vi "check_run_settings_dialog.vi"(0 "Enable":bool=TRUE, 2 "Current Run Settings":T1={"Operator"="", "Sample (or CRM) ID"="", "Sample Temp"=0.0, "Salinity"=0.0, "Sample Units"=FALSE, "Sample Size"=0.0, "Operation Mode"=TRUE}, 5 "error in (no error)":errorcluster) -> (15 "New Run Settings":T1={"Operator"="", "Sample (or CRM) ID"="", "Sample Temp"=0.0, "Salinity"=0.0, "Sample Units"=FALSE, "Sample Size"=0.0, "Operation Mode"=TRUE}, 18 "OK":bool, 19 "error out":errorcluster)   [LabVIEW 2010]
doc: "Displays a standard dialog box that prompts users to enter information, such as a user name and password.\n--------------------\n\nThis Express VI is configured as follows:\n\nMessage to Display to the User:\nThe inputs are:"
panel:
  out "String":string
  in  "Cancel":bool
  in  "OK2":bool
  in  "OK1":bool
  # "Please verify that the following settings are correct and update them if need be (especially Operation Mode and Sample Size)"
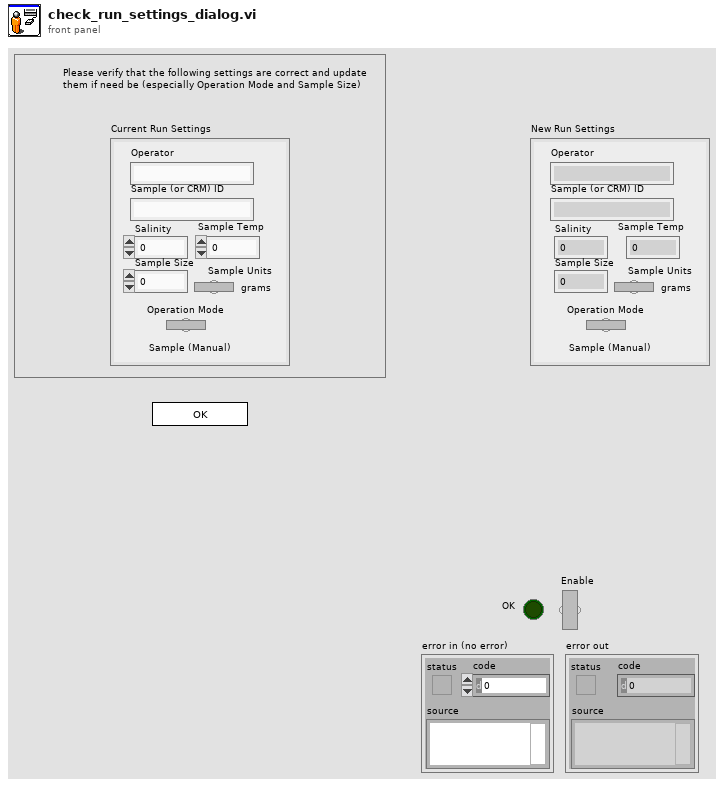
[diagram p1: front panel]
types:
  T1 = cluster{"Operator":string, "Sample (or CRM) ID":string, "Sample Temp":dbl, "Salinity":dbl, "Sample Units":bool, "Sample Size":dbl, "Operation Mode":bool}
  T2 = cluster{"Input Name":string, "Input Data Type":i32}[]
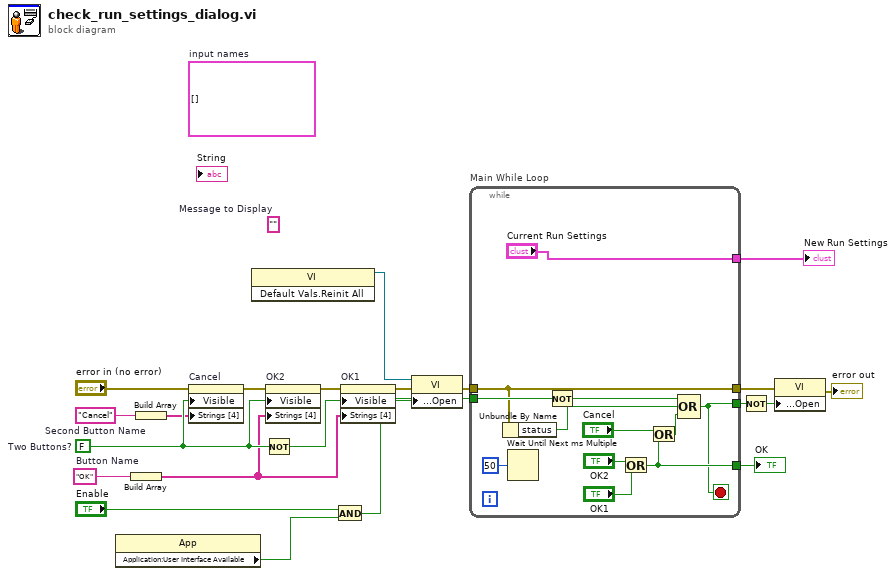
[diagram p0: block diagram]
diagram:
  (unwired) T2 []  # input names
  w13 = "Cancel"  # Second Button Name
  w11 = "OK"  # Button Name
  (unwired) ""  # Message to Display
  w21 = FALSE  # Two Buttons?
  n1 = property class="App"() -> ("Application:User Interface Available"=w3:bool)  [unwired: 2 in, 2 out]
  n2 = Build Array(w11) -> (w12:string[])
  n3 = Build Array(w13) -> (w14:string[])
  n4 = property on="Cancel" class="Bool"(error in="error in (no error)", "Visible"=w21, "Strings [4]"=w14) -> (error out=w18:errorcluster)  [unwired: 1 in, 1 out]
  n5 = invoke class="VI" method="Default Vals.Reinit All"() -> (reference out=w2:refnum<vi>)  [unwired: 3 in, 2 out]
  n6 = Not(x=w21) -> (.not. x?=w19:bool)
  n7 = property on="OK2" class="Bool"(error in=w18, "Visible"=w21, "Strings [4]"=w12) -> (error out=w17:errorcluster)  [unwired: 1 in, 1 out]
  n8 = And(x="Enable", y=w3) -> (x .and. y?=w4:bool)
  n9 = property on="OK1" class="Bool"(error in=w17, "Visible"=w19, "Strings [4]"=w12) -> (error out=w10:errorcluster)  [unwired: 1 in, 1 out]
  n10 = property class="VI"(reference=w2, error in=w10, "Front Panel Window:Open"=w4) -> (error out=w9:errorcluster)  [unwired: 1 out]
  n11 = while "Main While Loop" {
    tunnel: [w30] -> w20
    tunnel: w4 -> [w28]
    tunnel: [w26] -> w15
    tunnel: w9 -> [w25]
    tunnel: [w25] -> w7
    tunnel: ["Current Run Settings"] -> w1
    stop <- w26 stop-if-true
    n12 = Unbundle By Name(w25) -> ("status"=w23:bool)
    n13 = Wait Until Next ms Multiple(millisecond multiple=u32 50) -> ()  [unwired: 1 out]
    n14 = Not(x=w28) -> (.not. x?=w27:bool)
    n15 = Or(x="OK2", y="OK1") -> (x .or. y?=w30:bool)
    n16 = Or(x="Cancel", y=w30) -> (x .or. y?=w24:bool)
    n17 = Compound Arithmetic op=OR(w27, w23, w24) -> (w26:bool)
  }
  "OK" <- w20
  "New Run Settings" <- w1
  n18 = Not(x=w15) -> (.not. x?=w16:bool)
  n19 = property class="VI"(error in=w7, "Front Panel Window:Open"=w16) -> (error out=→"error out":errorcluster)  [unwired: 1 in, 1 out]
